vi "Read Controllers.vi"   [LabVIEW 2014]
uses:
  Begin/Global RefNums.vi
  <vilib>/Rock Robotics/WPI/Joystick/WPI_JoystickGetSetRefNum.vi
  Begin/Global Variables.vi
  <vilib>/Rock Robotics/Network Tables/SD Write Number.vi
types:
  T1 = typedef "WPI_JoystickDevRef.ctl" = cluster{"Device":T2}
  T2 = typedef "WPI_JoystickDeviceEnum.ctl" = enum16{"USB 0", "USB 1", "USB 2", "USB 3", "USB 4", "USB 5"}
  T3 = cluster{"Axes[0]":dbl, "Axes[1]":dbl, "Axes[2]":dbl, "Axes[3]":dbl, "Axes[4]":dbl, "Axes[5]":dbl, "Axes[6]":dbl, "Axes[7]":dbl, "Axes[8]":dbl}
  T4 = cluster{"Buttons[0]":bool, "Buttons[1]":bool, "Buttons[2]":bool, "Buttons[3]":bool, "Buttons[4]":bool, "Buttons[5]":bool, "Buttons[6]":bool, "Buttons[7]":bool, "Buttons[8]":bool}
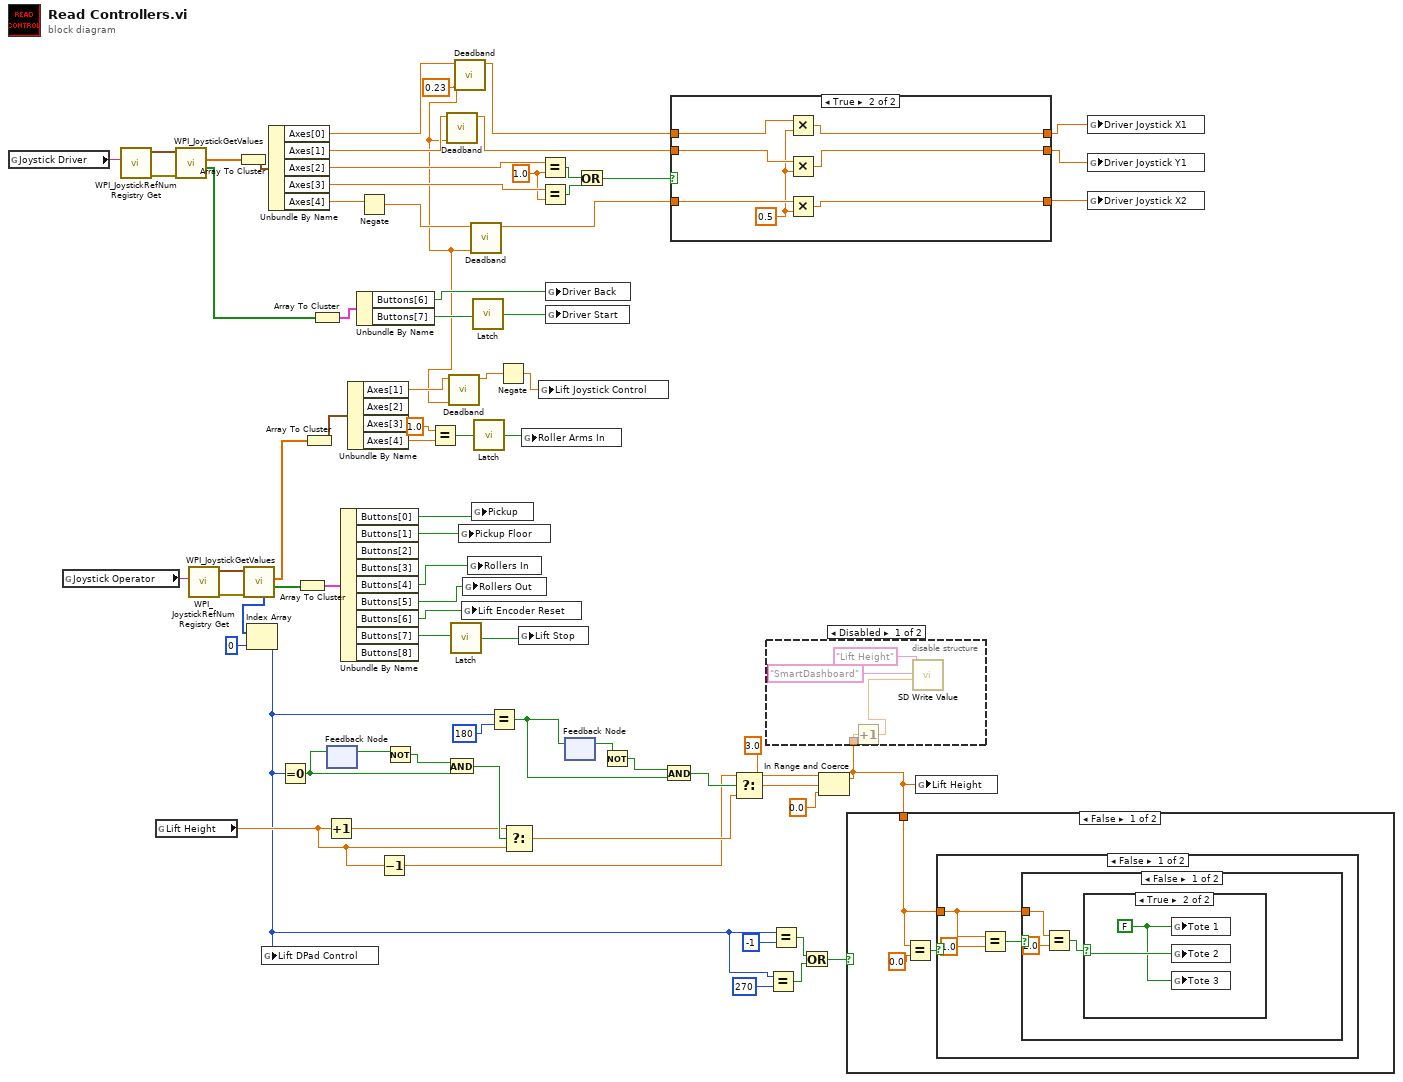
[diagram p0: block diagram]
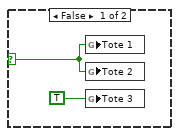
[diagram p2: hidden frame]
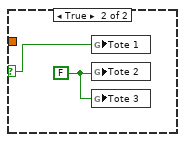
[diagram p3: hidden frame]
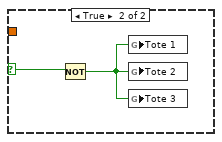
[diagram p4: hidden frame]
diagram:
  w9 = 0.23 ("Value to Deadband (default of 0.1)")
  w57 = 1.0 ("y")
  n1 = global read "Global RefNums.vi" "Joystick Driver"() -> (w73:string)
  n2 = global read "Global RefNums.vi" "Joystick Operator"() -> (w68:string)
  n3 = call <vilib>:"WPI_JoystickRefNum Registry Get.vi"("refnum name"=w73) -> ("error out"=w71:errorcluster, "JoystickDevRef"=w72:T1)  [unwired: 9 in]
  n4 = global read "Global Variables.vi" "Lift Height"() -> (w30:dbl)
  n5 = call <vilib>:"WPI_JoystickGetValues.vi"("error in (no error)"=w71, "JoystickDevRef"=w72) -> ("Buttons"=w56:bool[], "Axes"=w67:dbl[])  [unwired: 5 in, 3 out]
  n6 = call <vilib>:"WPI_JoystickRefNum Registry Get.vi"("refnum name"=w68) -> ("error out"=w70:errorcluster, "JoystickDevRef"=w69:T1)  [unwired: 9 in]
  n7 = Array To Cluster(array=w67) -> (cluster=w66:T3)
  n8 = call <vilib>:"WPI_JoystickGetValues.vi"("error in (no error)"=w70, "JoystickDevRef"=w69) -> ("Buttons"=w49:bool[], "Axes"=w19:dbl[], "POVs"=w43:i16[])  [unwired: 5 in, 2 out]
  n9 = Index Array(array=w43, index=0) -> (element=w2:i16)
  n10 = global write "Global Variables.vi" "Lift DPad Control"(w2) -> ()
  n11 = Unbundle By Name(w66) -> ("Axes[0]"=w50:dbl, "Axes[1]"=w53:dbl, "Axes[2]"=w62:dbl, "Axes[3]"=w58:dbl, "Axes[4]"=w25:dbl)
  n12 = Equal To 0?(x=w2) -> (x = 0?=w39:bool)
  n13 = Array To Cluster(array=w49) -> (cluster=w48:T4)
  n14 = Array To Cluster(array=w19) -> (cluster=w18:T3)
  n15 = Array To Cluster(array=w56) -> (cluster=w55:T4)
  n16 = Increment(x=w30) -> (x+1=w37:dbl)
  n17 = feedback-in #1(w39) -> ()
  n18 = feedback #1() -> (w41:bool)  [unwired: 1 in]
  n19 = Unbundle By Name(w48) -> ("Buttons[0]"=w47:bool, "Buttons[1]"=w46:bool, "Buttons[4]"=w13:bool, "Buttons[5]"=w12:bool, "Buttons[6]"=w11:bool, "Buttons[7]"=w45:bool)  [unwired: 3 out]
  n20 = Unbundle By Name(w18) -> ("Axes[1]"=w10:dbl, "Axes[4]"=w17:dbl)  [unwired: 2 out]
  n21 = Unbundle By Name(w55) -> ("Buttons[6]"=w21:bool, "Buttons[7]"=w23:bool)
  n22 = Negate(x=w25) -> (-x=w24:dbl)
  n23 = Decrement(x=w30) -> (x-1=w29:dbl)
  n24 = Not(x=w41) -> (.not. x?=w40:bool)
  n25 = Equal?(x=1.0, y=w17) -> (x = y?=w16:bool)
  n26 = call "Deadband.vi"("Value to Deadband (default of 0.1)"=w9, "Value"=w53) -> ("Deadbanded Value"=w52:dbl)  [unwired: 9 in]
  n27 = And(x=w40, y=w39) -> (x .and. y?=w38:bool)
  n28 = call "Deadband.vi"("Value to Deadband (default of 0.1)"=w9, "Value"=w10) -> ("Deadbanded Value"=w7:dbl)  [unwired: 9 in]
  n29 = call "Latch.vi"("Input"=w45) -> ("Output"=w44:bool)
  n30 = call "Deadband.vi"("Value to Deadband (default of 0.1)"=w9, "Value"=w50) -> ("Deadbanded Value"=w54:dbl)  [unwired: 9 in]
  n31 = global write "Global Variables.vi" "Pickup Floor"(w46) -> ()
  n32 = global write "Global Variables.vi" "Lift Encoder Reset"(w11) -> ()
  n33 = global write "Global Variables.vi" "Rollers Out"(w12) -> ()
  n34 = global write "Global Variables.vi" "Rollers In"(w13) -> ()
  n35 = call "Deadband.vi"("Value to Deadband (default of 0.1)"=w9, "Value"=w24) -> ("Deadbanded Value"=w51:dbl)  [unwired: 9 in]
  n36 = global write "Global Variables.vi" "Pickup"(w47) -> ()
  n37 = call "Latch.vi"("Input"=w23) -> ("Output"=w22:bool)
  n38 = call "Latch.vi"("Input"=w16) -> ("Output"=w15:bool)
  n39 = Equal?(x=w2, y=i16 180) -> (x = y?=w35:bool)
  n40 = Negate(x=w7) -> (-x=w6:dbl)
  n41 = Select(t=w37, s=w38, f=w30) -> (s? t:f=w31:dbl)
  n42 = global write "Global Variables.vi" "Lift Stop"(w44) -> ()
  n43 = global write "Global Variables.vi" "Roller Arms In"(w15) -> ()
  n44 = global write "Global Variables.vi" "Lift Joystick Control"(w6) -> ()
  n45 = Equal?(x=w62, y=w57) -> (x = y?=w60:bool)
  n46 = Equal?(x=w58, y=w57) -> (x = y?=w59:bool)
  n47 = global write "Global Variables.vi" "Driver Back"(w21) -> ()
  n48 = global write "Global Variables.vi" "Driver Start"(w22) -> ()
  n49 = feedback #2() -> (w34:bool)  [unwired: 1 in]
  n50 = feedback-in #2(w35) -> ()
  n51 = Or(x=w60, y=w59) -> (x .or. y?=w61:bool)
  n52 = Not(x=w34) -> (.not. x?=w33:bool)
  n53 = And(x=w33, y=w35) -> (x .and. y?=w32:bool)
  n54 = case shown="True" w61 {
    tunnel: w54 -> [w74 w83]
    tunnel: w52 -> [w75 w82]
    tunnel: w51 -> [w76 w81]
    tunnel: [w76 w77] -> w64
    tunnel: [w75 w78] -> w63
    tunnel: [w74 w79] -> w65
    frame False {
    }
    frame True {
      w80 = 0.5 ("y")
      n55 = Multiply(x=w83, y=w80) -> (x*y=w79:dbl)
      n56 = Multiply(x=w82, y=w80) -> (x*y=w78:dbl)
      n57 = Multiply(x=w81, y=w80) -> (x*y=w77:dbl)
    }
  }
  n58 = Select(t=w29, s=w32, f=w31) -> (s? t:f=w26:dbl)
  n59 = Equal?(x=w2, y=i16 270) -> (x = y?=w3:bool)
  n60 = Equal?(x=w2, y=i16 -1) -> (x = y?=w5:bool)
  n61 = Or(x=w5, y=w3) -> (x .or. y?=w1:bool)
  n62 = In Range and Coerce(upper limit=3.0, x=w26, lower limit=0.0) -> (coerced(x)=w20:dbl)  [unwired: 1 out]
  n63 = disable-structure shown="Disabled" {
    disable-tunnel: w20 -> [w85 _]
    frame Disabled {
      n64 = Increment(x=w85) -> (x+1=w84:dbl)
      n65 = call-poly <vilib>:"SD Write Value.vi"("Numeric"=w84, "Table Prefix"="SmartDashboard", "Name"="Lift Height") -> ()  [unwired: 7 in, 2 out]
    }
    frame Enabled {
    }
  }
  n66 = case shown="False" w1 {
    tunnel: w20 -> [w90 _]
    frame False {
      n67 = Equal?(x=w90, y=0.0) -> (x = y?=w89:bool)
      n68 = case shown="False" w89 {
        selector: w89 -> [_ w104]
        tunnel: w90 -> [w91 _]
        frame False {
          n69 = Equal?(x=w91, y=1.0) -> (x = y?=w92:bool)
          n70 = case shown="False" w92 {
            selector: w92 -> [_ w101]
            tunnel: w91 -> [w96 _]
            frame False {
              n71 = Equal?(x=w96, y=2.0) -> (x = y?=w94:bool)
              n72 = case shown="True" w94 {
                selector: w94 -> [w97 w100]
                frame False {
                  n73 = global write "Global Variables.vi" "Tote 1"(w97) -> ()
                  n74 = global write "Global Variables.vi" "Tote 2"(w97) -> ()
                  n75 = global write "Global Variables.vi" "Tote 3"(TRUE ("Tote 2")) -> ()
                }
                frame True {
                  w99 = FALSE ("Tote 0")
                  n76 = global write "Global Variables.vi" "Tote 1"(w99) -> ()
                  n77 = global write "Global Variables.vi" "Tote 2"(w100) -> ()
                  n78 = global write "Global Variables.vi" "Tote 3"(w99) -> ()
                }
              }
            }
            frame True {
              w102 = FALSE ("Tote 1")
              n79 = global write "Global Variables.vi" "Tote 1"(w101) -> ()
              n80 = global write "Global Variables.vi" "Tote 2"(w102) -> ()
              n81 = global write "Global Variables.vi" "Tote 3"(w102) -> ()
            }
          }
        }
        frame True {
          n82 = Not(x=w104) -> (.not. x?=w103:bool)
          n83 = global write "Global Variables.vi" "Tote 1"(w103) -> ()
          n84 = global write "Global Variables.vi" "Tote 2"(w103) -> ()
          n85 = global write "Global Variables.vi" "Tote 3"(w103) -> ()
        }
      }
    }
    frame True {
    }
  }
  n86 = global write "Global Variables.vi" "Lift Height"(w20) -> ()
  n87 = global write "Global Variables.vi" "Driver Joystick X1"(w65) -> ()
  n88 = global write "Global Variables.vi" "Driver Joystick Y1"(w63) -> ()
  n89 = global write "Global Variables.vi" "Driver Joystick X2"(w64) -> ()
